vi "PH_PSDBWriter.evt call write PSDB.vi"(0 "i ref in":refnum<vi>, 5 "error in (no error)":errorcluster) -> (14 "i ref out":refnum<vi>, 19 "error out":errorcluster)   [LabVIEW 2014, in "PH_PSDBWriter.lvlib"]
doc: "This VI sends a move out command"
uses:
  PH_PSDBWriter.lvlib
  CSCore/BaseProcess/BaseProcess.lvlib
  CSCore/CSSystem/CSSystemLib/CSSystemLib.lvlib
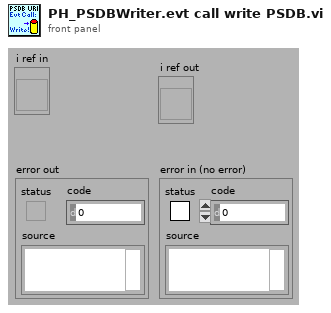
[diagram p1: front panel]
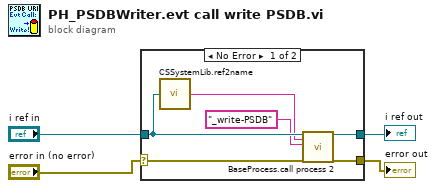
[diagram p0: block diagram]
diagram:
  n1 = case shown="No Error" "error in (no error)" {
    selector: "error in (no error)" -> [w7 w11]
    tunnel: [w10 w12] -> w2
    tunnel: [w9 w11] -> w1
    tunnel: "i ref in" -> [w8 w12]
    frame No Error {
      n2 = call "CSSystemLib.ref2name.vi"("obj refnum"=w8) -> ("name"=w5:string)
      n3 = call "BaseProcess.call process 2.vi"("i ref in"=w8, "Object"=w5, "Selector"="_write-PSDB", "error in (no error)"=w7) -> ("i ref out"=w10:refnum<vi>, "error out"=w9:errorcluster)  [unwired: 14 in]
    }
    frame Error {
    }
  }
  "error out" <- w1
  "i ref out" <- w2
